vi "FestoCPX.Station.Revolver.GetID.vi"(8 "error in":errorcluster) -> (0 "error out":errorcluster, 1 "ForkID":u8, 2 "RevID":T1 caption="RevolverID")   [LabVIEW 2016]
uses:
  FestoCPX.Station.RevolverID.ctl
  FestoCPX.DI.Signal.ctl
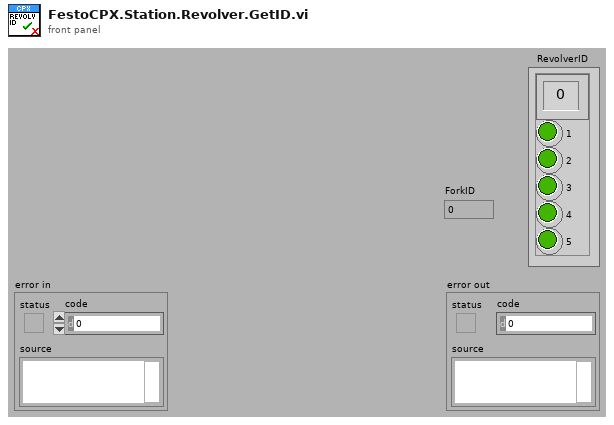
[diagram p1: front panel]
types:
  T1 = typedef "FestoCPX.Station.RevolverID.ctl" = cluster{"ID":u8, "1":bool, "2":bool, "3":bool, "4":bool, "5":bool}
  T2 = typedef "FestoCPX.DI.Signal.ctl" = enum16{"S.C. Emergency Stop", "S.C. Side Door Close", "S.C. Front Door Close", "S.C. Front Door Secured", "Button Start", "Button Stop", "Button Control", "Product Move Home", "Product Move Work", "Table Position", "Table Lock", "Product Lift A Home", "Product Lift B Home", "Product Arm OK", "Product Arm NOK", "Product Arm Work", "Revolver ID 1", "Revolver ID 2", "Revolver ID 3", "Revolver ID 4", "Revolver ID 5", "Air Pressure Inside", "Air Pressure Inlet", "Product Slot 1 A Present", "Product Slot 1 B Present", "Product Slot 2 A Present", "Product Slot 2 B Present", "Product Slot 3 A Present", "Product Slot 3 B Present", "Product Slot 4 A Present", "Product Slot 4 B Present", "Product Final A Present", "Product Final B Present", "Product Output A Present", "Product Output B Present", "Product Container OK Present", "Product Container NOK Present", "Fork ID 1", "Fork ID 2"}
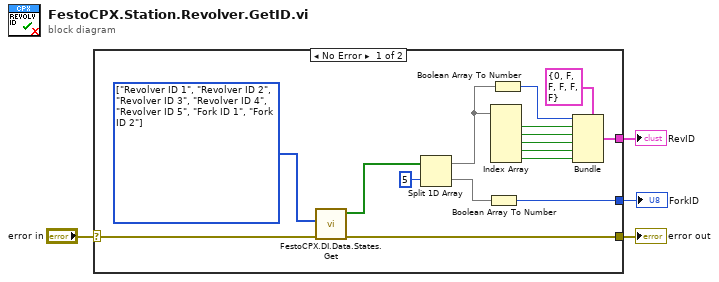
[diagram p0: block diagram]
diagram:
  n1 = case shown="No Error" "error in" {
    selector: "error in" -> [w20 w21]
    tunnel: [w19 w21] -> w4
    tunnel: [w12 _] -> w2
    tunnel: [w6 _] -> w1
    frame No Error {
      w18 = T2[] [enum."Revolver ID 1", enum."Revolver ID 2", enum."Revolver ID 3", enum."Revolver ID 4", enum."Revolver ID 5", enum."Fork ID 1", enum."Fork ID 2"] items=["S.C. Emergency Stop", "S.C. Side Door Close", "S.C. Front Door Close", "S.C. Front Door Secured", "Button Start", "Button Stop", "Button Control", "Product Move Home", "Product Move Work", "Table Position", "Table Lock", "Product Lift A Home", "Product Lift B Home", "Product Arm OK", "Product Arm NOK", "Product Arm Work", "Revolver ID 1", "Revolver ID 2", "Revolver ID 3", "Revolver ID 4", "Revolver ID 5", "Air Pressure Inside", "Air Pressure Inlet", "Product Slot 1 A Present", "Product Slot 1 B Present", "Product Slot 2 A Present", "Product Slot 2 B Present", "Product Slot 3 A Present", "Product Slot 3 B Present", "Product Slot 4 A Present", "Product Slot 4 B Present", "Product Final A Present", "Product Final B Present", "Product Output A Present", "Product Output B Present", "Product Container OK Present", "Product Container NOK Present", "Fork ID 1", "Fork ID 2"] ("CPX.DO")
      n2 = call "FestoCPX.DI.Data.States.Get.vi"("error in (no error)"=w20, "CPX.DI"=w18) -> ("error out"=w19:errorcluster, "State"=w5:bool[])  [unwired: 5 in, 3 out]
      n3 = Split 1D Array(array=w5, index=5) -> (first subarray=w8:bool[], second subarray=w7:bool[])
      n4 = Boolean Array To Number(Boolean array=w7) -> (number=w6:u32)
      n5 = Index Array(array=w8) -> (element #1=w11:bool, element #2=w16:bool, element #3=w15:bool, element #4=w14:bool, element #5=w13:bool)  [unwired: 5 in]
      n6 = Boolean Array To Number(Boolean array=w8) -> (number=w10:u32)
      n7 = Bundle(cluster=T1 {"ID"=0, "1"=FALSE, "2"=FALSE, "3"=FALSE, "4"=FALSE, "5"=FALSE} ("RevolverID"), "ID"=w10, "1"=w11, "2"=w16, "3"=w15, "4"=w14, "5"=w13) -> (w12:T1)
    }
    frame Error {
    }
  }
  "error out" <- w4
  "RevID" <- w2
  "ForkID" <- w1
